vi "HFRR ADV v014 new software.vi"() -> ()   [LabVIEW 2025] (continued)
    n917 = local read "Print 3"() -> (w1079:bool)
    n918 = Equal?(x=w1076, y=path "") -> (x = y?=w1075:bool)
    n919 = Not(x=w1075) -> (.not. x?=w1074:bool)
    n920 = property on="Print 3" class="Bool (strict)"("Visible"=w1074) -> ()  [unwired: 2 in, 2 out]
    n921 = case shown="True" w1079 {
      frame False {
        n922 = local write "Rd"(TRUE ("Boolean 7")) -> ()
      }
      frame True {
        n923 = flat-sequence {
          tunnel: [w1119] -> w1087
          tunnel: [w1106] -> w1085
          tunnel: [w1116] -> w1081
          tunnel: w1087 -> [w1128]
          tunnel: [w1128] -> w1086
          tunnel: w1085 -> [w1127]
          tunnel: [w1127] -> w1084
          tunnel: [w1125] -> w1083
          tunnel: [w1124] -> w1082
          tunnel: w1081 -> [w1124]
          tunnel: w1086 -> [w1130]
          tunnel: w1084 -> [w1131]
          tunnel: w1083 -> [_]
          tunnel: w1082 -> [w1129]
          frame #0 {
            n924 = case shown="True" "Rd" {
              frame False {
              }
              frame True {
                n925 = while {
                  tunnel: "abcdefABCDEF" ("string 2") -> [w1098]
                  shift-right: [w1096] -> w1090
                  shift-left: "" -> [w1095]
                  i -> [w1105]
                  stop <- w1104 stop-if-true
                  n926 = Random Number (0-1)() -> (number: 0 to 1=w1099:dbl)
                  n927 = Multiply(x=w1099, y=62.0) -> (x*y=w1101:dbl)
                  n928 = Decrement(x="Length 2") -> (x-1=w1094:i16)
                  n929 = To Word Integer(number=w1101) -> (16bit integer=w1102:i16)
                  n930 = String Subset(string=w1098, offset (0)=w1102, length (rest)=1 ("length (rest)")) -> (substring=w1097:string)
                  n931 = Greater Or Equal?(x=w1105, y=w1094) -> (x >= y?=w1104:bool)
                  n932 = Concatenate Strings(w1097, w1095) -> (w1096:string)
                }
                "String 10" <- w1090
                n933 = local write "Rd"(FALSE ("Boolean 7")) -> ()
              }
            }
          }
          frame #1 {
            w1117 = "_resized.jpg" ("command line")
            (unwired) ".jpg -resize 320x240 " ("string")
            (unwired) "Choose an Image File" ("prompt")
            # "-resize 1798x425"
            n934 = local read "Image Path"() -> (w1111:path)
            n935 = Strip Path(path=w1111) -> (stripped path=w1106:path, name=w1107:string)
            n936 = Match Pattern(string=w1107, regular expression=".jpg") -> (before substring=→"before substring 2":string, after substring=→"after substring":string)  [unwired: 1 in, 2 out]
            n937 = Match Pattern(string=w1107, regular expression="\\") -> (before substring=w1113:string)  [unwired: 1 in, 3 out]
            n938 = Match Pattern(string=w1113, regular expression=".jpg") -> (before substring=w1112:string)  [unwired: 1 in, 3 out]
            n939 = Concatenate Strings("cmd /c convert " ("string"), w1112, ".jpg -resize 320x240  " ("command line"), w1112, w1117) -> (w1120:string)
            n940 = call <vilib>:"System Exec.vi"("run minimized? (F)"=TRUE, "wait until completion? (T)"=TRUE, "working directory"=w1106, "command line"=w1120) -> ("error out"=w1119:errorcluster)  [unwired: 4 in, 3 out]
            "error out 2" <- w1119
            n941 = Concatenate Strings(w1112, w1117) -> (w1116:string)
          }
          frame #2 {
            n942 = Wait (ms)(milliseconds to wait=u32 2000 ("millisecond timer value")) -> (millisecond timer value=w1125:u32)
          }
          frame #3 {
            n943 = case shown="No Error" w1130 {
              tunnel: w1131 -> [w1134 _]
              tunnel: w1129 -> [w1132 _]
              frame No Error {
                (unwired) ".jpg" ("string")
                n944 = Path To String(path=w1134) -> (string=w1138:string)
                n945 = Concatenate Strings(w1138, "\\" ("string"), w1132) -> (w1137:string)
                n946 = String To Path(string=w1137) -> (path=w1136:path)
                n947 = call <vilib>:"Read JPEG File.vi"("path to JPEG file"=w1136) -> ("image data"=w1140:T16)  [unwired: 8 in, 2 out]
                "image data" <- w1140
                n948 = local write "Print 3"(FALSE ("Print 2")) -> ()
                n949 = call <vilib>:"Draw Flattened Pixmap.vi"("image data"=w1140) -> ("new picture"=→"new picture":picture)  [unwired: 8 in]
              }
              frame Error {
              }
            }
          }
        }
      }
    }
    n950 = Wait (ms)(milliseconds to wait=u32 20 ("millisecond timer value")) -> ()  [unwired: 1 out]
    n951 = local read "Quit"() -> (w1073:bool)
  }
  n952 = while {
    tunnel: w33 -> [_]
    tunnel: w17 -> [_]
    stop <- w1171 stop-if-true
    # "New Adv Logics"
    n953 = local read "Main Tab"() -> (w1151:T2)
    n954 = local read "Main Tab"() -> (w1169:T2)
    n955 = local read "Sign In"() -> (w1168:bool)
    n956 = case shown="\"Adv Scar\"" w1151 {
      frame "HOME", Default {
        n957 = local read "LIVE FEED MIN TEMP"() -> (w1304:bool)
        n958 = local write "LIVE FEED MAX TEMP"(TRUE ("LIVE FEED MAX TEMP")) -> ()
        n959 = local read "CAMERA ROI MIN TEMP"() -> (w1302:bool)
        n960 = case shown="True" w1304 {
          selector: w1304 -> [_ w1311]
          frame False {
          }
          frame True {
            n961 = Not(x=w1311) -> (.not. x?=w1310:bool)
            n962 = local write "LIVE FEED MIN TEMP"(w1310) -> ()
            n963 = call "CAMERA LIVE FEED FGV.vi"("Enum - Menu"=CAMERA_LIVE_FEED_ENUM."CAMERA MINIMIZE") -> ()  [unwired: 9 in, 2 out]
          }
        }
        n964 = case shown="True" w1302 {
          selector: w1302 -> [_ w1308]
          frame False {
          }
          frame True {
            n965 = Not(x=w1308) -> (.not. x?=w1307:bool)
            n966 = local write "CAMERA ROI MIN TEMP"(w1307) -> ()
            n967 = call "IMAGE ANALYSIS.vi"("Enum"=POST_ANALYSIS_ENUM."MINIMIZE UI") -> ()  [unwired: 9 in, 2 out]
          }
        }
        n968 = local write "CAMERA ROI MAX TEMP"(TRUE ("CAMERA ROI MAX TEMP")) -> ()
      }
      frame "Test Setup" {
        n969 = local read "LIVE FEED MIN TEMP"() -> (w1314:bool)
        n970 = local read "CAMERA ROI MIN TEMP"() -> (w1312:bool)
        n971 = local write "LIVE FEED MAX TEMP"(TRUE ("LIVE FEED MAX TEMP")) -> ()
        n972 = case shown="True" w1314 {
          selector: w1314 -> [_ w1321]
          frame False {
          }
          frame True {
            n973 = Not(x=w1321) -> (.not. x?=w1320:bool)
            n974 = local write "LIVE FEED MIN TEMP"(w1320) -> ()
            n975 = call "CAMERA LIVE FEED FGV.vi"("Enum - Menu"=CAMERA_LIVE_FEED_ENUM."CAMERA MINIMIZE") -> ()  [unwired: 9 in, 2 out]
          }
        }
        n976 = case shown="True" w1312 {
          selector: w1312 -> [_ w1318]
          frame False {
          }
          frame True {
            n977 = Not(x=w1318) -> (.not. x?=w1317:bool)
            n978 = local write "CAMERA ROI MIN TEMP"(w1317) -> ()
            n979 = call "IMAGE ANALYSIS.vi"("Enum"=POST_ANALYSIS_ENUM."MINIMIZE UI") -> ()  [unwired: 9 in, 2 out]
          }
        }
        n980 = local write "CAMERA ROI MAX TEMP"(TRUE ("CAMERA ROI MAX TEMP")) -> ()
      }
      frame "Acquire" {
        n981 = local read "LIVE FEED MIN TEMP"() -> (w1324:bool)
        n982 = local write "LIVE FEED MAX TEMP"(TRUE ("LIVE FEED MAX TEMP")) -> ()
        n983 = local read "CAMERA ROI MIN TEMP"() -> (w1322:bool)
        n984 = case shown="True" w1324 {
          selector: w1324 -> [_ w1331]
          frame False {
          }
          frame True {
            n985 = Not(x=w1331) -> (.not. x?=w1330:bool)
            n986 = local write "LIVE FEED MIN TEMP"(w1330) -> ()
            n987 = call "CAMERA LIVE FEED FGV.vi"("Enum - Menu"=CAMERA_LIVE_FEED_ENUM."CAMERA MINIMIZE") -> ()  [unwired: 9 in, 2 out]
          }
        }
        n988 = case shown="True" w1322 {
          selector: w1322 -> [_ w1328]
          frame False {
          }
          frame True {
            n989 = Not(x=w1328) -> (.not. x?=w1327:bool)
            n990 = local write "CAMERA ROI MIN TEMP"(w1327) -> ()
            n991 = call "IMAGE ANALYSIS.vi"("Enum"=POST_ANALYSIS_ENUM."MINIMIZE UI") -> ()  [unwired: 9 in, 2 out]
          }
        }
        n992 = local write "CAMERA ROI MAX TEMP"(TRUE ("CAMERA ROI MAX TEMP")) -> ()
      }
      frame "Adv Scar" {
        n993 = local read "CAMERA ROI MIN TEMP"() -> (w1332:bool)
        n994 = case shown="True" "LIVE FEED MAX TEMP" {
          selector: "LIVE FEED MAX TEMP" -> [_ w1353]
          frame False {
          }
          frame True {
            n995 = Not(x=w1353) -> (.not. x?=w1352:bool)
            n996 = local write "LIVE FEED MAX TEMP"(w1352) -> ()
            n997 = call "CAMERA LIVE FEED FGV.vi"("Enum - Menu"=CAMERA_LIVE_FEED_ENUM."CAMERA RESTORE") -> ("error out"=w1343:errorcluster)  [unwired: 9 in, 1 out]
            n998 = Type Cast(type=30, x=0) -> (*(type *) &x=w1347:i32)
            n999 = Add(x=w1347, y=48) -> (x+y=w1348:i32)
            n1000 = call "CAMERA LIVE FEED FGV.vi"("Enum - Menu"=CAMERA_LIVE_FEED_ENUM."CAMERA MODE SET", "error in (no error)"=w1343, "CAMERA MODE"=w1348) -> ("error out"=w1340:errorcluster)  [unwired: 7 in, 1 out]
            n1001 = call "CAMERA LIVE FEED FGV.vi"("Enum - Menu"=CAMERA_LIVE_FEED_ENUM."CAMERA GRAY", "error in (no error)"=w1340) -> ("error out"=w1339:errorcluster)  [unwired: 8 in, 1 out]
            n1002 = call "LIST FILE NAMES.vi"("error in (no error)"=w1339) -> ("error out"=w1349:errorcluster, "filenames"=w1350:string[])  [unwired: 9 in]
            n1003 = property on="FILE 3" class="CmbBox"(error in=w1349, "Strings[]"=w1350) -> ()  [unwired: 1 in, 2 out]
          }
        }
        n1004 = case shown="True" w1332 {
          selector: w1332 -> [_ w1338]
          frame False {
          }
          frame True {
            n1005 = Not(x=w1338) -> (.not. x?=w1337:bool)
            n1006 = local write "CAMERA ROI MIN TEMP"(w1337) -> ()
            n1007 = call "IMAGE ANALYSIS.vi"("Enum"=POST_ANALYSIS_ENUM."MINIMIZE UI") -> ()  [unwired: 9 in, 2 out]
          }
        }
        n1008 = local write "CAMERA ROI MAX TEMP"(TRUE ("CAMERA ROI MAX TEMP")) -> ()
        "LIVE FEED MIN TEMP" <- TRUE ("LIVE FEED MIN TEMP")
      }
      frame "Adv Scar Report" {
        n1009 = local read "CAMERA ROI MAX TEMP"() -> (w1354:bool)
        n1010 = local read "LIVE FEED MIN TEMP"() -> (w1356:bool)
        n1011 = local write "LIVE FEED MAX TEMP"(TRUE ("LIVE FEED MAX TEMP")) -> ()
        n1012 = case shown="True" w1356 {
          selector: w1356 -> [_ w1365]
          frame False {
          }
          frame True {
            n1013 = Not(x=w1365) -> (.not. x?=w1364:bool)
            n1014 = local write "LIVE FEED MIN TEMP"(w1364) -> ()
            n1015 = call "CAMERA LIVE FEED FGV.vi"("Enum - Menu"=CAMERA_LIVE_FEED_ENUM."CAMERA MINIMIZE") -> ()  [unwired: 9 in, 2 out]
          }
        }
        n1016 = case shown="True" w1354 {
          selector: w1354 -> [_ w1362]
          frame False {
          }
          frame True {
            n1017 = Not(x=w1362) -> (.not. x?=w1360:bool)
            n1018 = local write "CAMERA ROI MAX TEMP"(w1360) -> ()
            n1019 = call "IMAGE ANALYSIS.vi"("Enum"=POST_ANALYSIS_ENUM."SHOW UI") -> ("error out"=w1359:errorcluster)  [unwired: 9 in, 1 out]
            n1020 = call "LIST FILE NAMES.vi"("error in (no error)"=w1359) -> ("filenames"=w1358:string[])  [unwired: 9 in, 1 out]
            n1021 = property on="Test File List :" class="CmbBox"("Strings[]"=w1358) -> ()  [unwired: 2 in, 2 out]
          }
        }
        n1022 = local write "CAMERA ROI MIN TEMP"(TRUE ("CAMERA ROI MIN TEMP")) -> ()
      }
      frame "Compare Files" {
        n1023 = local read "LIVE FEED MIN TEMP"() -> (w1368:bool)
        n1024 = local write "LIVE FEED MAX TEMP"(TRUE ("LIVE FEED MAX TEMP")) -> ()
        n1025 = local read "CAMERA ROI MIN TEMP"() -> (w1366:bool)
        n1026 = case shown="True" w1368 {
          selector: w1368 -> [_ w1375]
          frame False {
          }
          frame True {
            n1027 = Not(x=w1375) -> (.not. x?=w1374:bool)
            n1028 = local write "LIVE FEED MIN TEMP"(w1374) -> ()
            n1029 = call "CAMERA LIVE FEED FGV.vi"("Enum - Menu"=CAMERA_LIVE_FEED_ENUM."CAMERA MINIMIZE") -> ()  [unwired: 9 in, 2 out]
          }
        }
        n1030 = case shown="True" w1366 {
          selector: w1366 -> [_ w1372]
          frame False {
          }
          frame True {
            n1031 = Not(x=w1372) -> (.not. x?=w1371:bool)
            n1032 = local write "CAMERA ROI MIN TEMP"(w1371) -> ()
            n1033 = call "IMAGE ANALYSIS.vi"("Enum"=POST_ANALYSIS_ENUM."MINIMIZE UI") -> ()  [unwired: 9 in, 2 out]
          }
        }
        n1034 = local write "CAMERA ROI MAX TEMP"(TRUE ("CAMERA ROI MAX TEMP")) -> ()
      }
      frame "About" {
        n1035 = local read "LIVE FEED MIN TEMP"() -> (w1378:bool)
        n1036 = local write "LIVE FEED MAX TEMP"(TRUE ("LIVE FEED MAX TEMP")) -> ()
        n1037 = local read "CAMERA ROI MIN TEMP"() -> (w1377:bool)
        n1038 = case shown="True" w1378 {
          selector: w1378 -> [_ w1385]
          frame False {
          }
          frame True {
            n1039 = Not(x=w1385) -> (.not. x?=w1384:bool)
            n1040 = local write "LIVE FEED MIN TEMP"(w1384) -> ()
            n1041 = call "CAMERA LIVE FEED FGV.vi"("Enum - Menu"=CAMERA_LIVE_FEED_ENUM."CAMERA MINIMIZE") -> ()  [unwired: 9 in, 2 out]
          }
        }
        n1042 = case shown="True" w1377 {
          selector: w1377 -> [_ w1382]
          frame False {
          }
          frame True {
            n1043 = Not(x=w1382) -> (.not. x?=w1381:bool)
            n1044 = local write "CAMERA ROI MIN TEMP"(w1381) -> ()
            n1045 = call "IMAGE ANALYSIS.vi"("Enum"=POST_ANALYSIS_ENUM."MINIMIZE UI") -> ()  [unwired: 9 in, 2 out]
          }
        }
        n1046 = local write "CAMERA ROI MAX TEMP"(TRUE ("CAMERA ROI MIN TEMP")) -> ()
      }
      frame "Advance" {
        n1047 = local read "LIVE FEED MIN TEMP"() -> (w1388:bool)
        n1048 = local write "LIVE FEED MAX TEMP"(TRUE ("LIVE FEED MAX TEMP")) -> ()
        n1049 = local read "CAMERA ROI MIN TEMP"() -> (w1386:bool)
        n1050 = case shown="True" w1388 {
          selector: w1388 -> [_ w1395]
          frame False {
          }
          frame True {
            n1051 = Not(x=w1395) -> (.not. x?=w1394:bool)
            n1052 = local write "LIVE FEED MIN TEMP"(w1394) -> ()
            n1053 = call "CAMERA LIVE FEED FGV.vi"("Enum - Menu"=CAMERA_LIVE_FEED_ENUM."CAMERA MINIMIZE") -> ()  [unwired: 9 in, 2 out]
          }
        }
        n1054 = local write "CAMERA ROI MAX TEMP"(TRUE ("CAMERA ROI MAX TEMP")) -> ()
        n1055 = case shown="True" w1386 {
          selector: w1386 -> [_ w1392]
          frame False {
          }
          frame True {
            n1056 = Not(x=w1392) -> (.not. x?=w1391:bool)
            n1057 = local write "CAMERA ROI MIN TEMP"(w1391) -> ()
            n1058 = call "IMAGE ANALYSIS.vi"("Enum"=POST_ANALYSIS_ENUM."MINIMIZE UI") -> ()  [unwired: 9 in, 2 out]
          }
        }
      }
      frame "Mooha" {
        n1059 = local read "LIVE FEED MIN TEMP"() -> (w1398:bool)
        n1060 = local write "LIVE FEED MAX TEMP"(TRUE ("LIVE FEED MAX TEMP")) -> ()
        n1061 = local read "CAMERA ROI MIN TEMP"() -> (w1396:bool)
        n1062 = case shown="True" w1398 {
          selector: w1398 -> [_ w1405]
          frame False {
          }
          frame True {
            n1063 = Not(x=w1405) -> (.not. x?=w1404:bool)
            n1064 = local write "LIVE FEED MIN TEMP"(w1404) -> ()
            n1065 = call "CAMERA LIVE FEED FGV.vi"("Enum - Menu"=CAMERA_LIVE_FEED_ENUM."CAMERA MINIMIZE") -> ()  [unwired: 9 in, 2 out]
          }
        }
        n1066 = local write "CAMERA ROI MAX TEMP"(TRUE ("CAMERA ROI MAX TEMP")) -> ()
        n1067 = case shown="True" w1396 {
          selector: w1396 -> [_ w1402]
          frame False {
          }
          frame True {
            n1068 = Not(x=w1402) -> (.not. x?=w1401:bool)
            n1069 = local write "CAMERA ROI MIN TEMP"(w1401) -> ()
            n1070 = call "IMAGE ANALYSIS.vi"("Enum"=POST_ANALYSIS_ENUM."MINIMIZE UI") -> ()  [unwired: 9 in, 2 out]
          }
        }
      }
    }
    n1071 = local read "Auto Start Test"() -> (w1142:bool)
    n1072 = case shown="True" "sign in temp" {
      frame False {
      }
      frame True {
        w1178 = 1 ("y")
        n1073 = local read "USERNAME"() -> (w1184:string)
        n1074 = local read "USER ID"() -> (w1181:string)
        n1075 = call <vilib>:"Trim Whitespace.vi"("string"=w1184) -> ("trimmed string"=w1183:string)  [unwired: 1 in]
        n1076 = call <vilib>:"Trim Whitespace.vi"("string"=w1181) -> ("trimmed string"=w1182:string)  [unwired: 1 in]
        n1077 = String Length(string=w1183) -> (length=w1180:i32)
        n1078 = String Length(string=w1182) -> (length=w1179:i32)
        n1079 = Greater?(x=w1180, y=w1178) -> (0:w1177:bool)
        n1080 = Greater?(x=w1179, y=w1178) -> (0:w1176:bool)
        n1081 = And(x=w1177, y=w1176) -> (x .and. y?=w1175:bool)
        n1082 = case shown="True" w1175 {
          frame False {
            n1083 = property on="Sign In" class="Bool (strict)"("DisabledEnum"=T18."Disabled" ("Disabled")) -> ()  [unwired: 2 in, 2 out]
          }
          frame True {
            n1084 = property on="Sign In" class="Bool (strict)"("DisabledEnum"=T18."Enabled" ("Disabled")) -> ()  [unwired: 2 in, 2 out]
          }
        }
      }
    }
    n1085 = local read "Air Temperature"() -> (w1159:bool)
    n1086 = local read "Coefficient Of Friction"() -> (w1160:bool)
    n1087 = case shown="False" w1142 {
      frame False {
        n1088 = local read "Auto stop temp"() -> (w1172:bool)
        n1089 = case shown="True" w1172 {
          frame False {
          }
          frame True {
            n1090 = local write "Auto Start Temp"(FALSE ("Auto Start Temp")) -> ()
          }
        }
      }
      frame True {
        "Auto stop temp" <- TRUE ("Auto stop temp")
      }
    }
    n1091 = local read "Humidity"() -> (w1158:bool)
    n1092 = case shown="\"HOME\"" w1169 {
      frame "HOME" {
        n1093 = local write "main tab sub"(enum32{"Page 1", "Page 2"}."Page 1" ("main tab sub")) -> ()
      }
      frame Default {
        n1094 = local write "main tab sub"(enum32{"Page 1", "Page 2"}."Page 2" ("main tab sub")) -> ()
      }
    }
    n1095 = case shown="True" w1168 {
      selector: w1168 -> [_ w1519]
      frame False {
      }
      frame True {
        n1096 = Not(x=w1519) -> (.not. x?=w1518:bool)
        n1097 = local write "Sign In"(w1518) -> ()
        n1098 = local write "Main Dashboard Buttons"(T24."Test Setup" ("Main Dashboard Buttons")) -> ()
      }
    }
    n1099 = case shown="\"Numeric Display\", Default" "Num/Graph" {
      frame "Numeric Display", Default {
        n1100 = property on="Single/Multiple" class="RadioBtnsControl (strict)"("Visible"=FALSE) -> ()  [unwired: 2 in, 2 out]
        n1101 = property on="Single - Graph" class="Ring (strict)"("Visible"=FALSE) -> ()  [unwired: 2 in, 2 out]
        n1102 = local write "Main Tab Display"(T4."Dashboard 1" ("Main Tab Display")) -> ()
      }
      frame "Graph Display" {
        n1103 = property on="Single/Multiple" class="RadioBtnsControl (strict)"("Visible"=TRUE) -> ()  [unwired: 2 in, 2 out]
        n1104 = case shown="\"Multiple\"" "Single/Multiple" {
          frame "Single ", Default {
            n1105 = property on="Single - Graph" class="Ring (strict)"("Visible"=TRUE) -> ()  [unwired: 2 in, 2 out]
            n1106 = local write "Main Tab Display"(T4."Dashboard 3" ("Main Tab Display")) -> ()
          }
          frame "Multiple" {
            n1107 = property on="Single - Graph" class="Ring (strict)"("Visible"=FALSE) -> ()  [unwired: 2 in, 2 out]
            n1108 = local write "Main Tab Display"(T4."Dashboard 2" ("Main Tab Display")) -> ()
          }
        }
      }
    }
    n1109 = local read "Stroke"() -> (w1157:bool)
    n1110 = local read "USERNAME"() -> (w1163:string)
    n1111 = local read "USER ID"() -> (w1162:string)
    n1112 = case shown="True" w1160 {
      selector: w1160 -> [_ w1445]
      frame False {
      }
      frame True {
        n1113 = Not(x=w1445) -> (.not. x?=w1444:bool)
        n1114 = local write "Coefficient Of Friction"(w1444) -> ()
        n1115 = local write "Tab Control 2"(T6."Coefficient Of Friction" ("Tab Control 2")) -> ()
      }
    }
    n1116 = case shown="True" w1159 {
      selector: w1159 -> [_ w1442]
      frame False {
      }
      frame True {
        n1117 = Not(x=w1442) -> (.not. x?=w1440:bool)
        n1118 = local write "Air Temperature"(w1440) -> ()
        n1119 = local write "Tab Control 2"(T6."Air Temperature" ("Tab Control 2")) -> ()
      }
    }
    n1120 = local write "Operator ID"(w1162) -> ()
    n1121 = case shown="True" w1157 {
      selector: w1157 -> [_ w1436]
      frame False {
      }
      frame True {
        n1122 = Not(x=w1436) -> (.not. x?=w1434:bool)
        n1123 = local write "Stroke"(w1434) -> ()
        n1124 = local write "Tab Control 2"(T6."Stroke" ("Tab Control 2")) -> ()
      }
    }
    n1125 = local write "tested by"(w1163) -> ()
    n1126 = case shown="True" w1158 {
      selector: w1158 -> [_ w1439]
      frame False {
      }
      frame True {
        n1127 = Not(x=w1439) -> (.not. x?=w1437:bool)
        n1128 = local write "Humidity"(w1437) -> ()
        n1129 = local write "Tab Control 2"(T6."Humidity" ("Tab Control 2")) -> ()
      }
    }
    n1130 = case shown="\"Calibration\"" "Main Dashboard Buttons" {
      tunnel: [T2."HOME" ("Main Tab") T2."Test Setup" ("Main Tab") T2."Acquire" ("Main Tab") T2."Adv Scar" ("Main Tab") T2."Adv Scar Report" ("Main Tab") T2."Compare Files" ("Main Tab") T2."Calibration" ("Main Tab") T2."About" ("Main Tab") T2."Advance" ("Main Tab")] -> w1141
      frame "Home", Default {
      }
      frame "Test Setup" {
      }
      frame "Dashboard" {
      }
      frame "Imaging" {
      }
      frame "Report" {
      }
      frame "Analysis" {
      }
      frame "Calibration" {
      }
      frame "About" {
      }
      frame "Advance" {
      }
    }
    n1131 = Wait (ms)(milliseconds to wait=u32 100) -> ()  [unwired: 1 out]
    n1132 = local read "Main Tab Display"() -> (w1161:T4)
    n1133 = local write "Main Tab"(w1141) -> ()
    n1134 = case shown="\"Dashboard 3\"" w1161 {
      frame "Dashboard 1", Default {
        n1135 = property on="Reset Graph" class="Bool (strict)"("Visible"=FALSE) -> ()  [unwired: 2 in, 2 out]
      }
      frame "Dashboard 2" {
        n1136 = property on="Reset Graph" class="Bool (strict)"("Visible"=TRUE) -> ()  [unwired: 2 in, 2 out]
      }
      frame "Dashboard 3" {
        n1137 = property on="Reset Graph" class="Bool (strict)"("Visible"=TRUE) -> ()  [unwired: 2 in, 2 out]
      }
    }
    n1138 = local read "SCAR MEASURMENT"() -> (w1149:enum32{"Auto Scar", "Manual Scar"})
    n1139 = local read "Humidity"() -> (w1164:bool)
    n1140 = local read "Cap Live Image"() -> (w1146:bool)
    n1141 = local read "Sample Temperature"() -> (w1156:bool)
    n1142 = local read "Air Temp vs Humidity"() -> (w1154:bool)
    n1143 = local read "Frequency"() -> (w1155:bool)
    n1144 = case shown="True" w1164 {
      frame False {
        n1145 = local write "Humidity On Command"(TRUE ("Humidity On Command")) -> ()
        n1146 = case shown="True" "Humidity Off Command" {
          selector: "Humidity Off Command" -> [_ w1452]
          frame False {
          }
          frame True {
            n1147 = stacked-sequence {
              frame #0 {
                n1148 = local read "WriteHumidity"() -> (w1454:string[])
                n1149 = Insert Into Array(array=w1454, new element="R;1" ("new element/subarray")) -> (w1455:string[])  [unwired: 1 in]
                n1150 = local write "WriteHumidity"(w1455) -> ()
              }
              frame #1 {
                n1151 = Wait (ms)(milliseconds to wait=u32 2000) -> ()  [unwired: 1 out]
              }
              frame #2 {
                n1152 = local read "EVENT LOG"() -> (w1461:string)
                n1153 = local read "WriteHumidity"() -> (w1458:string[])
                n1154 = call "Event Log.vi"("Content"="Humidity Control Off" ("string"), "EVENT LOG"=w1461) -> ("EVENT LOG"=w1462:string)  [unwired: 8 in, 1 out]
                n1155 = local write "EVENT LOG"(w1462) -> ()
                n1156 = Insert Into Array(array=w1458, new element="R;1" ("new element/subarray")) -> (w1459:string[])  [unwired: 1 in]
                n1157 = local write "WriteHumidity"(w1459) -> ()
              }
            }
            n1158 = Not(x=w1452) -> (.not. x?=w1451:bool)
            n1159 = local write "Humidity Off Command"(w1451) -> ()
          }
        }
      }
      frame True {
        n1160 = local write "Humidity Off Command"(TRUE ("Humidity Off Command")) -> ()
        n1161 = case shown="True" "Humidity On Command" {
          selector: "Humidity On Command" -> [_ w1466]
          frame False {
          }
          frame True {
            n1162 = stacked-sequence {
              frame #0 {
                n1163 = local read "Set Rh"() -> (w1472:dbl)
                n1164 = Number To Fractional String(number=w1472, precision (6)=i16 2) -> (F-format string=w1473:string)  [unwired: 2 in]
                n1165 = local read "WriteHumidity"() -> (w1470:string[])
                n1166 = Concatenate Strings("M;" ("new element/subarray"), w1473) -> (w1471:string)
                n1167 = Insert Into Array(array=w1470, new element=w1471) -> (w1469:string[])  [unwired: 1 in]
                n1168 = local write "WriteHumidity"(w1469) -> ()
              }
              frame #1 {
                n1169 = Wait (ms)(milliseconds to wait=u32 2000) -> ()  [unwired: 1 out]
              }
              frame #2 {
                n1170 = local read "Set Rh"() -> (w1480:dbl)
                n1171 = Number To Fractional String(number=w1480, precision (6)=i16 2) -> (F-format string=w1481:string)  [unwired: 2 in]
                n1172 = local read "WriteHumidity"() -> (w1478:string[])
                n1173 = Concatenate Strings("M;" ("new element/subarray"), w1481) -> (w1479:string)
                n1174 = Insert Into Array(array=w1478, new element=w1479) -> (w1477:string[])  [unwired: 1 in]
                n1175 = local write "WriteHumidity"(w1477) -> ()
              }
              frame #3 {
                n1176 = Wait (ms)(milliseconds to wait=u32 1500) -> ()  [unwired: 1 out]
              }
              frame #4 {
                (unwired) "% RH" ("string")
                (unwired) i16 2 ("precision (6)")
                (unwired) "M;" ("new element/subarray")
                n1177 = local read "Set Rh"() -> (w1488:dbl)
                n1178 = Number To Fractional String(number=w1488, precision (6)=i16 2) -> (F-format string=w1485:string)  [unwired: 2 in]
                n1179 = local read "WriteHumidity"() -> (w1490:string[])
                n1180 = Concatenate Strings("M;" ("new element/subarray"), w1485) -> (w1489:string)
                n1181 = Concatenate Strings("Humidity Set to : " ("string"), w1485, "% RH" ("string")) -> (w1483:string)
                n1182 = Insert Into Array(array=w1490, new element=w1489) -> (w1491:string[])  [unwired: 1 in]
                n1183 = disable-structure shown="Enabled" {
                  frame Enabled {
                    n1184 = local read "EVENT LOG"() -> (w1494:string)
                    n1185 = call "Event Log.vi"("Content"="Humidity Control On", "EVENT LOG"=w1494) -> ("EVENT LOG"=w1495:string)  [unwired: 8 in, 1 out]
                    n1186 = local write "EVENT LOG"(w1495) -> ()
                  }
                  frame Disabled {
                  }
                }
                n1187 = disable-structure shown="Enabled" {
                  disable-tunnel: w1483 -> [_ _]
                  frame Enabled {
                    n1188 = local read "EVENT LOG"() -> (w1497:string)
                    n1189 = call "Event Log.vi"("Content"="Humidity Control On", "EVENT LOG"=w1497) -> ("EVENT LOG"=w1498:string)  [unwired: 8 in, 1 out]
                    n1190 = local write "EVENT LOG"(w1498) -> ()
                  }
                  frame Disabled {
                  }
                }
                n1191 = local write "WriteHumidity"(w1491) -> ()
              }
            }
            n1192 = Not(x=w1466) -> (.not. x?=w1465:bool)
            n1193 = local write "Humidity On Command"(w1465) -> ()
          }
        }
      }
    }
    n1194 = Equal?(x=w1149, y=enum32{"Auto Scar", "Manual Scar"}."Auto Scar" ("SCAR MEASURMENT")) -> (x = y?=w1145:bool)
    n1195 = local read "TEST STANDARD"() -> (w1152:T3)
    n1196 = And(x=w1146, y=w1145) -> (x .and. y?=w1147:bool)
    n1197 = case shown="True" w1147 {
      selector: w1147 -> [_ w1251]
      tunnel: errorcluster {"status"=FALSE, "code"=0, "source"=""} ("error in (no error) 3") -> [_ w1252]
      frame False {
      }
      frame True {
        n1198 = stacked-sequence {
          tunnel: w1252 -> [_ _ _ _ _ _ _ w1300]
          tunnel: w1251 -> [_ _ _ _ _ w1281 _ _]
          frame #0 {
            n1199 = call "CAMERA LIVE FEED FGV.vi"("Enum - Menu"=CAMERA_LIVE_FEED_ENUM."CAMERA MINIMIZE") -> ()  [unwired: 9 in, 2 out]
          }
          frame #1 {
            n1200 = property on="Auto Scar Check  2" class="Clust (strict)"("Visible"=TRUE) -> ()  [unwired: 2 in, 2 out]
          }
          frame #2 {
            n1201 = String To Path(string="C:\\LAB-IQ\\Image Calibrate v01.dcf") -> (path=w1257:path)
            n1202 = Open/Create/Replace File ("Open File")(file path (use dialog)=w1257) -> (refnum out=w1258:refnum<file>)  [unwired: 5 in, 2 out]
            n1203 = for {
              N: 4 -> [_]
              tunnel: w1258 -> [w1264]
              i -> [w1260]
              n1204 = Read from Text File ("Read File")(file (use dialog)=w1264) -> (text=w1265:string)  [unwired: 3 in, 3 out]
              n1205 = String Subset(string=w1265, offset (0)=6, length (rest)=10 ("length (rest)")) -> (substring=w1261:string)
              n1206 = Fract/Exp String To Number(string=w1261) -> (number=w1259:dbl)  [unwired: 3 in, 1 out]
              n1207 = case shown="0" w1260 {
                tunnel: w1259 -> [w1266 w1267 _ w1268 _]
                frame 0 {
                  "5x Gain" <- w1266
                }
                frame 1 {
                  "10x Gain" <- w1267
                }
                frame 2 {
                }
                frame 3 {
                  "100x gain" <- w1268
                }
                frame 4, Default {
                }
              }
            }
          }
          frame #3 {
            n1208 = local read "FILE 3"() -> (w1274:string)
            n1209 = call <vilib>:"Trim Whitespace.vi"("string"="C:\\LAB-IQ\\images\\") -> ("trimmed string"=w1276:string)  [unwired: 1 in]
            n1210 = String To Path(string=w1276) -> (path=w1275:path)
            n1211 = Concatenate Strings(w1274, ".png" ("string")) -> (w1273:string)
            n1212 = Build Path(base path=w1275, name or relative path=w1273) -> (appended path=w1271:path)
            "Image path" <- w1271
            n1213 = Path To String(path=w1271) -> (string=w1270:string)
            n1214 = call "CAMERA LIVE FEED FGV.vi"("Enum - Menu"=CAMERA_LIVE_FEED_ENUM."CAMERA SAVE", "Image Path"=w1270) -> ()  [unwired: 8 in, 2 out]
          }
          frame #4 {
            n1215 = One Button Dialog(message="Image saved successfully") -> ()  [unwired: 1 in, 1 out]
          }
          frame #5 {
            n1216 = local read "TEST STANDARD"() -> (w1280:T3)
            n1217 = local read "Magnification len live scar"() -> (w1292:string)
            n1218 = Not(x=w1281) -> (.not. x?=w1282:bool)
            n1219 = local write "Cap Live Image"(w1282) -> ()
            n1220 = case shown="\"ISO 12156\"" w1280 {
              tunnel: ["ASTM D6079" "ISO 12156"] -> w1279
              frame "ASTM D6079", Default {
              }
              frame "ISO 12156" {
              }
            }
            n1221 = case shown="\"5x\", Default" w1292 {
              tunnel: [w1295 w1296] -> w1291
              frame "5x", Default {
                n1222 = local read "5x Gain"() -> (w1295:dbl)
              }
              frame "10x" {
                # "5x"
                n1223 = local read "10x Gain"() -> (w1296:dbl)
              }
            }
            n1224 = local read "Image path"() -> (w1290:path)
            n1225 = local read "FILE 3"() -> (w1283:string)
            n1226 = call "EDGE DETCTION.vi"("GAIN VALUE"=w1291, "Image Path"=w1290) -> ("error out"=w1289:errorcluster, "return value"=w1288:cluster{string, string, dbl, dbl, dbl})  [unwired: 8 in]
            n1227 = Bundle By Name(cluster=T25 {"File Name"="", "Test Method"="", "Operator"="", "Fuel Description"="", "Date and time"=""} ("Main Ref"), "File Name"=w1283, "Test Method"=w1279) -> (w1284:T25)
            n1228 = call "duf file read.vi"("error in (no error)"=w1289, "Main Ref"=w1284) -> ("error out"=w1287:errorcluster, "Main Ref 2"=w1285:T25)  [unwired: 8 in]
            n1229 = call "EDGE DETECTION REPORT.vi"("error in (no error)"=w1287, "return value 2"=w1288, "Main Ref"=w1285) -> ()  [unwired: 8 in, 1 out]
          }
          frame #6 {
            n1230 = property on="Auto Scar Check  2" class="Clust (strict)"("Visible"=FALSE) -> ()  [unwired: 2 in, 2 out]
          }
          frame #7 {
            n1231 = call "CAMERA LIVE FEED FGV.vi"("Enum - Menu"=CAMERA_LIVE_FEED_ENUM."CAMERA MINIMIZE", "error in (no error)"=w1300) -> ()  [unwired: 8 in, 2 out]
            n1232 = local write "Main Dashboard Buttons"(T1."Home" ("Main Dashboard Buttons")) -> ()
            n1233 = local write "Main Tab"(T2."HOME" ("Main Tab")) -> ()
          }
        }
      }
    }
    n1234 = local read "Heater Button"() -> (w1153:bool)
    n1235 = case shown="True" w1155 {
      selector: w1155 -> [_ w1430]
      frame False {
      }
      frame True {
        n1236 = Not(x=w1430) -> (.not. x?=w1428:bool)
        n1237 = local write "Frequency"(w1428) -> ()
        n1238 = local write "Tab Control 2"(T6."Frequency" ("Tab Control 2")) -> ()
      }
    }
    n1239 = case shown="True" w1154 {
      selector: w1154 -> [_ w1427]
      frame False {
      }
      frame True {
        n1240 = Not(x=w1427) -> (.not. x?=w1425:bool)
        n1241 = local write "Air Temp vs Humidity"(w1425) -> ()
        n1242 = local write "Tab Control 2"(T6."Air Temp vs Rh" ("Tab Control 2")) -> ()
      }
    }
    n1243 = case shown="True" w1156 {
      selector: w1156 -> [_ w1433]
      frame False {
      }
      frame True {
        n1244 = Not(x=w1433) -> (.not. x?=w1431:bool)
        n1245 = local write "Sample Temperature"(w1431) -> ()
        n1246 = local write "Tab Control 2"(T6."Sample Temperature" ("Tab Control 2")) -> ()
      }
    }
    n1247 = case shown="\"Custom\"" w1152 {
      frame "ASTM D6079", Default {
        w1406 = "ASTM D6079 TEST CONDITIONS" ("Standard 2")
        n1248 = local write "Standard 2"(w1406) -> ()
        n1249 = local write "Standard"(w1406) -> ()
      }
      frame "ISO 12156" {
        w1407 = "ISO 12156 TEST CONDITIONS" ("Standard 2")
        n1250 = local write "Standard 2"(w1407) -> ()
        n1251 = local write "Standard"(w1407) -> ()
      }
      frame "CEC F-096-A-06" {
        w1408 = "CEC F-096-A-06 TEST CONDITIONS" ("Standard 2")
        n1252 = local write "Standard 2"(w1408) -> ()
        n1253 = local write "Standard"(w1408) -> ()
      }
      frame "Custom" {
        w1409 = "CUSTOM TEST CONDITIONS" ("Standard 2")
        n1254 = local write "Standard 2"(w1409) -> ()
        n1255 = local write "Standard"(w1409) -> ()
      }
    }
    n1256 = case shown="True" w1153 {
      frame False {
        n1257 = local write "Temperature On Command"(TRUE ("Temperature On Command")) -> ()
        n1258 = case shown="True" "Temperature Off Command" {
          selector: "Temperature Off Command" -> [_ w1413]
          frame False {
          }
          frame True {
            n1259 = Not(x=w1413) -> (.not. x?=w1412:bool)
            n1260 = local read "EVENT LOG"() -> (w1416:string)
            n1261 = local write "Temperature Off Command"(w1412) -> ()
            n1262 = call "Event Log.vi"("Content"="Heater Off", "EVENT LOG"=w1416) -> ("EVENT LOG"=w1415:string)  [unwired: 8 in, 1 out]
            n1263 = local write "EVENT LOG"(w1415) -> ()
          }
        }
      }
      frame True {
        n1264 = local write "Temperature Off Command"(TRUE ("Temperature Off Command")) -> ()
        n1265 = case shown="True" "Temperature On Command" {
          selector: "Temperature On Command" -> [_ w1420]
          frame False {
          }
          frame True {
            n1266 = Not(x=w1420) -> (.not. x?=w1419:bool)
            n1267 = local write "Temperature On Command"(w1419) -> ()
            n1268 = disable-structure shown="Enabled" {
              disable-tunnel: "Heater On" -> [w1422 _]
              frame Enabled {
                n1269 = local read "EVENT LOG"() -> (w1423:string)
                n1270 = call "Event Log.vi"("Content"=w1422, "EVENT LOG"=w1423) -> ("EVENT LOG"=w1424:string)  [unwired: 8 in, 1 out]
                n1271 = local write "EVENT LOG"(w1424) -> ()
              }
              frame Disabled {
              }
            }
          }
        }
      }
    }
    n1272 = local read "Main Tab"() -> (w1144:T2)
    n1273 = case shown="\"About\"" w1144 {
      frame "HOME", Default {
        w1187 = T18."Enabled" ("Disabled")
        n1274 = local read "Service Password enable"() -> (w1189:bool)
        n1275 = property on="Imaging" class="Bool (strict)"("DisabledEnum"=w1187) -> ()  [unwired: 2 in, 2 out]
        n1276 = property on="Dashboard" class="Bool (strict)"("DisabledEnum"=w1187) -> ()  [unwired: 2 in, 2 out]
        n1277 = property on="Test Setup" class="Bool (strict)"("DisabledEnum"=w1187) -> ()  [unwired: 2 in, 2 out]
        n1278 = property on="Analysis" class="Bool (strict)"("DisabledEnum"=w1187) -> ()  [unwired: 2 in, 2 out]
        n1279 = property on="Home" class="Bool (strict)"("DisabledEnum"=w1187) -> ()  [unwired: 2 in, 2 out]
        n1280 = property on="Report" class="Bool (strict)"("DisabledEnum"=w1187) -> ()  [unwired: 2 in, 2 out]
        n1281 = property on="Main Dashboard Buttons" class="RadioBtnsControl (strict)"("DisabledEnum"=w1187) -> ()  [unwired: 2 in, 2 out]
        n1282 = property on="Calibration" class="Bool (strict)"("DisabledEnum"=w1187) -> ()  [unwired: 2 in, 2 out]
        n1283 = case shown="True" w1189 {
          tunnel: [T18."Disabled" ("Disabled") T18."Enabled" ("Disabled")] -> w1188
          frame False {
          }
          frame True {
          }
        }
        n1284 = property on="About" class="Bool (strict)"("DisabledEnum"=w1188) -> ()  [unwired: 2 in, 2 out]
      }
      frame "Test Setup" {
        w1194 = T18."Enabled" ("Disabled")
        n1285 = local read "Service Password enable"() -> (w1193:bool)
        n1286 = property on="Dashboard" class="Bool (strict)"("DisabledEnum"=T18."Disabled" ("Disabled")) -> ()  [unwired: 2 in, 2 out]
        n1287 = property on="Imaging" class="Bool (strict)"("DisabledEnum"=w1194) -> ()  [unwired: 2 in, 2 out]
        n1288 = property on="Analysis" class="Bool (strict)"("DisabledEnum"=w1194) -> ()  [unwired: 2 in, 2 out]
        n1289 = property on="Home" class="Bool (strict)"("DisabledEnum"=w1194) -> ()  [unwired: 2 in, 2 out]
        n1290 = property on="Report" class="Bool (strict)"("DisabledEnum"=w1194) -> ()  [unwired: 2 in, 2 out]
        n1291 = property on="Test Setup" class="Bool (strict)"("DisabledEnum"=w1194) -> ()  [unwired: 2 in, 2 out]
        n1292 = case shown="True" w1193 {
          tunnel: [T18."Disabled" ("Disabled") T18."Enabled" ("Disabled")] -> w1192
          frame False {
          }
          frame True {
          }
        }
        n1293 = property on="About" class="Bool (strict)"("DisabledEnum"=w1192) -> ()  [unwired: 2 in, 2 out]
      }
      frame "Adv Scar" {
        w1201 = T18."Enabled" ("Disabled")
        n1294 = property on="Dashboard" class="Bool (strict)"("DisabledEnum"=T18."Disabled" ("Disabled")) -> ()  [unwired: 2 in, 2 out]
        n1295 = property on="Imaging" class="Bool (strict)"("DisabledEnum"=w1201) -> ()  [unwired: 2 in, 2 out]
        n1296 = property on="Analysis" class="Bool (strict)"("DisabledEnum"=w1201) -> ()  [unwired: 2 in, 2 out]
        n1297 = property on="Home" class="Bool (strict)"("DisabledEnum"=w1201) -> ()  [unwired: 2 in, 2 out]
        n1298 = property on="Report" class="Bool (strict)"("DisabledEnum"=w1201) -> ()  [unwired: 2 in, 2 out]
        n1299 = property on="Test Setup" class="Bool (strict)"("DisabledEnum"=w1201) -> ()  [unwired: 2 in, 2 out]
        n1300 = local read "Service Password enable"() -> (w1199:bool)
        n1301 = case shown="True" w1199 {
          tunnel: [T18."Disabled" ("Disabled") T18."Enabled" ("Disabled")] -> w1198
          frame False {
          }
          frame True {
          }
        }
        n1302 = property on="About" class="Bool (strict)"("DisabledEnum"=w1198) -> ()  [unwired: 2 in, 2 out]
      }
      frame "Calibration" {
        w1204 = T18."Enabled" ("Disabled")
        n1303 = property on="Dashboard" class="Bool (strict)"("DisabledEnum"=T18."Disabled" ("Disabled")) -> ()  [unwired: 2 in, 2 out]
        n1304 = property on="Imaging" class="Bool (strict)"("DisabledEnum"=w1204) -> ()  [unwired: 2 in, 2 out]
        n1305 = property on="Analysis" class="Bool (strict)"("DisabledEnum"=w1204) -> ()  [unwired: 2 in, 2 out]
        n1306 = property on="Home" class="Bool (strict)"("DisabledEnum"=w1204) -> ()  [unwired: 2 in, 2 out]
        n1307 = property on="Report" class="Bool (strict)"("DisabledEnum"=w1204) -> ()  [unwired: 2 in, 2 out]
        n1308 = property on="Test Setup" class="Bool (strict)"("DisabledEnum"=w1204) -> ()  [unwired: 2 in, 2 out]
        n1309 = local read "Service Password enable"() -> (w1206:bool)
        n1310 = property on="Calibration" class="Bool (strict)"("DisabledEnum"=w1204) -> ()  [unwired: 2 in, 2 out]
        n1311 = case shown="True" w1206 {
          tunnel: [T18."Disabled" ("Disabled") T18."Enabled" ("Disabled")] -> w1205
          frame False {
          }
          frame True {
          }
        }
        n1312 = property on="About" class="Bool (strict)"("DisabledEnum"=w1205) -> ()  [unwired: 2 in, 2 out]
      }
      frame "Adv Scar Report" {
        w1212 = T18."Enabled" ("Disabled")
        n1313 = property on="Dashboard" class="Bool (strict)"("DisabledEnum"=T18."Disabled" ("Disabled")) -> ()  [unwired: 2 in, 2 out]
        n1314 = property on="Imaging" class="Bool (strict)"("DisabledEnum"=w1212) -> ()  [unwired: 2 in, 2 out]
        n1315 = property on="Analysis" class="Bool (strict)"("DisabledEnum"=w1212) -> ()  [unwired: 2 in, 2 out]
        n1316 = property on="Home" class="Bool (strict)"("DisabledEnum"=w1212) -> ()  [unwired: 2 in, 2 out]
        n1317 = property on="Report" class="Bool (strict)"("DisabledEnum"=w1212) -> ()  [unwired: 2 in, 2 out]
        n1318 = property on="Test Setup" class="Bool (strict)"("DisabledEnum"=w1212) -> ()  [unwired: 2 in, 2 out]
        n1319 = local read "Service Password enable"() -> (w1211:bool)
        n1320 = case shown="True" w1211 {
          tunnel: [T18."Disabled" ("Disabled") T18."Enabled" ("Disabled")] -> w1210
          frame False {
          }
          frame True {
          }
        }
        n1321 = property on="About" class="Bool (strict)"("DisabledEnum"=w1210) -> ()  [unwired: 2 in, 2 out]
      }
      frame "Compare Files" {
        w1218 = T18."Enabled" ("Disabled")
        n1322 = local read "Service Password enable"() -> (w1217:bool)
        n1323 = property on="Dashboard" class="Bool (strict)"("DisabledEnum"=T18."Disabled" ("Disabled")) -> ()  [unwired: 2 in, 2 out]
        n1324 = property on="Imaging" class="Bool (strict)"("DisabledEnum"=w1218) -> ()  [unwired: 2 in, 2 out]
        n1325 = property on="Analysis" class="Bool (strict)"("DisabledEnum"=w1218) -> ()  [unwired: 2 in, 2 out]
        n1326 = property on="Home" class="Bool (strict)"("DisabledEnum"=w1218) -> ()  [unwired: 2 in, 2 out]
        n1327 = property on="Report" class="Bool (strict)"("DisabledEnum"=w1218) -> ()  [unwired: 2 in, 2 out]
        n1328 = property on="Test Setup" class="Bool (strict)"("DisabledEnum"=w1218) -> ()  [unwired: 2 in, 2 out]
        n1329 = case shown="True" w1217 {
          tunnel: [T18."Disabled" ("Disabled") T18."Enabled" ("Disabled")] -> w1216
          frame False {
          }
          frame True {
          }
        }
        n1330 = property on="About" class="Bool (strict)"("DisabledEnum"=w1216) -> ()  [unwired: 2 in, 2 out]
      }
      frame "Acquire" {
        n1331 = local read "Service Password enable"() -> (w1223:bool)
        n1332 = property on="Test Setup" class="Bool (strict)"("DisabledEnum"=T18."Disabled" ("Disabled")) -> ()  [unwired: 2 in, 2 out]
        n1333 = local read "Auto Start Test"() -> (w1225:bool)
        n1334 = local read "RUN"() -> (w1227:bool)
        n1335 = case shown="True" w1223 {
          tunnel: [T18."Disabled" ("Disabled") T18."Enabled" ("Disabled")] -> w1224
          frame False {
          }
          frame True {
          }
        }
        n1336 = Or(x=w1227, y=w1225) -> (x .or. y?=w1226:bool)
        n1337 = case shown="True" w1226 {
          tunnel: [T18."Enabled" ("Disabled") T18."Disabled" ("Disabled")] -> w1222
          frame False {
          }
          frame True {
          }
        }
        n1338 = property on="About" class="Bool (strict)"("DisabledEnum"=w1224) -> ()  [unwired: 2 in, 2 out]
        n1339 = property on="Imaging" class="Bool (strict)"("DisabledEnum"=w1222) -> ()  [unwired: 2 in, 2 out]
        n1340 = property on="Dashboard" class="Bool (strict)"("DisabledEnum"=w1222) -> ()  [unwired: 2 in, 2 out]
        n1341 = property on="Analysis" class="Bool (strict)"("DisabledEnum"=w1222) -> ()  [unwired: 2 in, 2 out]
        n1342 = property on="Home" class="Bool (strict)"("DisabledEnum"=w1222) -> ()  [unwired: 2 in, 2 out]
        n1343 = property on="Report" class="Bool (strict)"("DisabledEnum"=w1222) -> ()  [unwired: 2 in, 2 out]
        n1344 = property on="Calibration" class="Bool (strict)"("DisabledEnum"=w1222) -> ()  [unwired: 2 in, 2 out]
      }
      frame "About" {
        n1345 = local read "FILE"() -> (w1241:string)
        n1346 = local read "TEST FILE NAM,E SAVED"() -> (w1234:bool)
        n1347 = call <vilib>:"Trim Whitespace.vi"("string"=w1241) -> ("trimmed string"=w1240:string)  [unwired: 1 in]
        n1348 = local read "Auto Start Test"() -> (w1244:bool)
        n1349 = String Length(string=w1240) -> (length=w1239:i32)
        n1350 = Greater?(x=w1239, y=1) -> (0:w1236:bool)
        n1351 = And(x=w1236, y=w1234) -> (x .and. y?=w1235:bool)
        n1352 = local read "RUN"() -> (w1246:bool)
        n1353 = case shown="True" w1235 {
          tunnel: [T18."Disabled" ("Disabled") T18."Enabled" ("Disabled")] -> w1237
          frame False {
          }
          frame True {
          }
        }
        n1354 = Or(x=w1246, y=w1244) -> (x .or. y?=w1245:bool)
        n1355 = property on="About" class="Bool (strict)"("DisabledEnum"=T18."Enabled" ("Disabled")) -> ()  [unwired: 2 in, 2 out]
        n1356 = case shown="False" w1245 {
          tunnel: [T18."Enabled" ("Disabled") T18."Disabled" ("Disabled")] -> w1243
          frame False {
          }
          frame True {
          }
        }
        n1357 = property on="Dashboard" class="Bool (strict)"("DisabledEnum"=w1237) -> ()  [unwired: 2 in, 2 out]
        n1358 = property on="Test Setup" class="Bool (strict)"("DisabledEnum"=T18."Disabled" ("Disabled")) -> ()  [unwired: 2 in, 2 out]
        n1359 = property on="Imaging" class="Bool (strict)"("DisabledEnum"=w1243) -> ()  [unwired: 2 in, 2 out]
        n1360 = property on="Analysis" class="Bool (strict)"("DisabledEnum"=w1243) -> ()  [unwired: 2 in, 2 out]
        n1361 = property on="Home" class="Bool (strict)"("DisabledEnum"=w1243) -> ()  [unwired: 2 in, 2 out]
        n1362 = property on="Report" class="Bool (strict)"("DisabledEnum"=w1243) -> ()  [unwired: 2 in, 2 out]
      }
    }
    n1363 = local read "Quit"() -> (w1171:bool)
    "Single" <- "Single - Graph"
  }
  n1364 = disable-structure shown="Disabled" {
    disable-tunnel: [w1523 _] -> w39
    disable-tunnel: _ -> [w1522 _]
    frame Disabled {
      n1365 = while {
        tunnel: w1522 -> [_]
        tunnel: [w1524] -> w1523
        tunnel: [w1525] -> _
        i -> [w1525]
        stop <- w1524 stop-if-true
        w1541 = u16 10 items=["1.0"=10, "1.5"=15, "2.0"=20] ("stop bits (10: 1 bit)")
        n1366 = Wait (ms)(milliseconds to wait=u32 10) -> ()  [unwired: 1 out]
        n1367 = call-poly "VISA Configure Serial Port"("VISA resource name"=refnum<visa-resource-name> "ASRL1::INSTR" ("COM PORT"), "timeout (10sec)"=u32 10, "baud rate (9600)"=u32 57600, "data bits (8)"=u16 8, "stop bits (10: 1 bit)"=w1541) -> ("VISA resource name out"=w1527:refnum<visa-resource-name>, "error out"=w1536:errorcluster)  [unwired: 9 in]
        n1368 = VISA Read(VISA resource name=w1527, byte count=u32 2 ("byte count (0)")) -> (read buffer=w1535:string)  [unwired: 1 in, 3 out]
        n1369 = String Subset(string=w1535, offset (0)=0, length (rest)=2 ("length (rest)")) -> (substring=w1534:string)
        n1370 = Match Pattern(string=w1534, regular expression="<>") -> (offset past match=w1531:i32)  [unwired: 1 in, 3 out]
        n1371 = Greater Or Equal?(x=w1531, y=0) -> (x >= y?=w1526:bool)
        n1372 = case shown="True" w1526 {
          tunnel: w1527 -> [_ w1545]
          tunnel: w1536 -> [_ w1544]
          frame False {
          }
          frame True {
            n1373 = VISA Read(VISA resource name=w1545, byte count=u32 32 ("byte count (0)"), error in (no error)=w1544) -> (read buffer=w1543:string)  [unwired: 3 out]
            n1374 = String Subset(string=w1543, offset (0)=0, length (rest)=8 ("length (rest)")) -> (substring=w1547:string)
            n1375 = String Subset(string=w1543, offset (0)=8, length (rest)=8 ("length (rest)")) -> (substring=w1548:string)
            n1376 = Decimal String To Number(string=w1548) -> (number=w1555:i32)  [unwired: 2 in, 1 out]
            n1377 = Decimal String To Number(string=w1547) -> (number=w1551:i32)  [unwired: 2 in, 1 out]
            n1378 = Divide(x=w1555, y=10000) -> ()  [unwired: 1 out]
            n1379 = Divide(x=w1551, y=1000000) -> ()  [unwired: 1 out]
          }
        }
        n1380 = local read "Quit"() -> (w1524:bool)
      }
    }
    frame Enabled {
    }
  }
  n1381 = while {
    shift-right: [w1570] -> w52
    shift-left: _ -> [w1561]
    shift-right: [w1569] -> w51
    shift-left: errorcluster {"status"=TRUE, "code"=0, "source"="Init"} ("error IO") -> [w1563]
    tunnel: [w1558] -> w42
    tunnel: [w1568] -> _
    i -> [w1568]
    stop <- w1558 stop-if-true
    n1382 = local read "Port 1a"() -> (w1564:bool)
    n1383 = local read "Port 3"() -> (w1565:bool)
    n1384 = local read "Com Port 1"() -> (w1562:refnum<visa-resource-name>)
    n1385 = Or(x=w1565, y=w1564) -> (x .or. y?=w1567:bool)
    n1386 = Unbundle(w1563) -> ("status"=→"Port 3":bool)  [unwired: 2 out]
    n1387 = Not Equal?(x=w1562, y=w1561) -> (x != y?=w1559:bool)
    n1388 = case shown="True" w1567 {
      frame False {
        w1573 = TRUE ("Visible")
        n1389 = property on="Port 1a" class="Bool (strict)"("Visible"=w1573) -> ()  [unwired: 2 in, 2 out]
        n1390 = property on="Port 3" class="Bool (strict)"("Visible"=w1573) -> ()  [unwired: 2 in, 2 out]
      }
      frame True {
        w1574 = TRUE ("Visible")
        n1391 = property on="Port 1a" class="Bool (strict)"("Visible"=w1574) -> ()  [unwired: 2 in, 2 out]
        n1392 = property on="Port 3" class="Bool (strict)"("Visible"=w1574) -> ()  [unwired: 2 in, 2 out]
      }
    }
    n1393 = Wait (ms)(milliseconds to wait=u32 40) -> ()  [unwired: 1 out]
    n1394 = case shown="True" w1559 {
      tunnel: [w1571 errorcluster {"status"=TRUE, "code"=0, "source"="Init"} ("error out")] -> w1560
      tunnel: w1563 -> [w1571 _]
      frame False {
      }
      frame True {
      }
    }
    n1395 = case shown="Error" w1560 {
      selector: w1560 -> [w1582 w1609]
      tunnel: [w1576 w1613] -> w1570
      tunnel: [w1584 w1607] -> w1569
      tunnel: w1561 -> [w1583 w1611]
      frame No Error {
        n1396 = property class="Instr"(reference=w1583, error in=w1582) -> (reference out=w1580:refnum<visa-resource-name>, error out=w1581:errorcluster, "Serial Settings:Number of Bytes at Serial Port"=w1577:u32)
        n1397 = Greater?(x=w1577, y=u32 5) -> (0:w1575:bool)
        n1398 = Not(x=w1575) -> (.not. x?=→"Port 1a":bool)
        n1399 = while {
          tunnel: [w1602] -> w1584
          tunnel: [w1601] -> w1585
          tunnel: w1581 -> [w1600]
          tunnel: w1580 -> [w1599]
          stop <- TRUE stop-if-true
          n1400 = property class="Instr" props=["Serial Settings:Number of Bytes at Serial Port"](reference=w1599, error in=w1600) -> (reference out=w1604:refnum<visa-resource-name>, error out=w1603:errorcluster)  [unwired: 1 out]
          n1401 = VISA Read(VISA resource name=w1604, byte count=u32 50, error in (no error)=w1603) -> (VISA resource name out=w1601:refnum<visa-resource-name>, read buffer=w1586:string, error out=w1602:errorcluster)  [unwired: 1 out]
          "UNI READ" <- w1586
          n1402 = Spreadsheet String To Array(delimiter (Tab)=";", format string="", spreadsheet string=w1586, array type (2D Dbl)=dbl[] []) -> (array=w1596:dbl[])
          n1403 = Index Array(array=w1596) -> (element #1=→"LVDT MIN":dbl, element #2=→"LVDT MAX":dbl, element #3=→"LVDT Peak":dbl, element #4=→"pizo raw":dbl, element #5=→"Friction":dbl, element #6=→"cof 2":dbl)  [unwired: 6 in]
        }
        n1404 = VISA Flush I/O Buffer(VISA resource name=w1585) -> (VISA resource name out=w1576:refnum<visa-resource-name>)  [unwired: 2 in, 1 out]
      }
      frame Error {
        w1619 = u16 0 items=["None", "XON/XOFF", "RTS/CTS", "XON/XOFF & RTS/CTS", "DTR/DSR", "XON/XOFF & DTR/DSR"] ("flow control (0:none)  2")
        w1617 = u16 10 items=["1.0"=10, "1.5"=15, "2.0"=20] ("stop bits 2")
        w1615 = u16 0 items=["None", "Odd", "Even", "Mark", "Space"] ("parity 2")
        w1616 = u32 10000  # timeout (10sec)
        n1405 = VISA Close(VISA resource name=w1611, error in (no error)=w1609) -> (error out=w1612:errorcluster)
        n1406 = local write "Port 1a"(FALSE ("Port 1a")) -> ()
        n1407 = local read "Com Port 1"() -> (w1606:refnum<visa-resource-name>)
        n1408 = call <vilib>:"Clear Errors.vi"("error in (no error)"=w1612) -> ("error out"=w1610:errorcluster)  [unwired: 5 in, 1 out]
        n1409 = call-poly "VISA Configure Serial Port"("VISA resource name"=w1606, "timeout (10sec)"=w1616, "baud rate (9600)"=u32 250000 ("baud rate  2"), "data bits (8)"=u16 8 ("data bits  2"), "parity (0:none)"=w1615, "error in (no error)"=w1610, "stop bits (10: 1 bit)"=w1617, "flow control (0:none)"=w1619) -> ("VISA resource name out"=w1620:refnum<visa-resource-name>, "error out"=w1621:errorcluster)  [unwired: 6 in]
        n1410 = flat-sequence {
          tunnel: w1620 -> [w1623]
          tunnel: w1621 -> [w1622]
          tunnel: [w1623] -> w1613
          tunnel: [w1622] -> w1607
          frame #0 {
            n1411 = Wait (ms)(milliseconds to wait=u32 50) -> ()  [unwired: 1 out]
          }
        }
        "Residual Uno" <- ""
        "Port 1 Error" <- w1607
      }
    }
    n1412 = local read "Quit"() -> (w1558:bool)
    "Error Uno" <- w1563
  }
  n1413 = while {
    stop <- w1633 stop-if-true
    # "V0OLTAGE TO STROKE (peice vise calibration)"
    n1414 = Wait (ms)(milliseconds to wait=u32 10) -> ()  [unwired: 1 out]
    n1415 = local read "LVDT Peak"() -> (w1625:dbl)
    n1416 = formula code="// Dynamic Parameterized Linear Interpolation Node\n// Inputs: vpp_val, voltages (Array), distances (Array)\n// Outputs: stroke\n\nint i = 0;\nint segments = 11; // 12 points make 11 interpolation segments\n\n// 1. Lower Boundary Clamp\nif (vpp_val <= voltages[0]) {\n    stroke = distances[0];\n}\n// 2. Upper Boundary Clamp\nelse if (vpp_val >= voltages[segments]) {\n    stroke = distances[segments];\n}\n// 3. Dynamic Segment Search Loop\nelse {\n    stroke = distances[0]; // Fallback baseline\n    for (i = 0; i < segments; i++) {\n        if (vpp_val >= voltages[i] && vpp_val <= voltages[i+1]) {\n            // Standard linear interpolation formula using array lookups\n            stroke = distances[i] + (vpp_val - voltages[i]) * (distances[i+1] - distances[i]) / (voltages[i+1] - voltages[i]);\n            break; // Segment found, safely exit the loop\n        }\n    }\n}"("vpp_val"=w1625, "voltages"="calibration values", "distances"="STROKE") -> ("stroke"=→"LVDT STROKE":dbl)
    n1417 = local read "Calibration Tare Value"() -> (w1629:dbl)
    n1418 = local read "Calibration Tare"() -> (w1627:bool)
    n1419 = Subtract(x=w1625, y=w1629) -> (x-y=→"LVDT STROKE  Calibration":dbl)
    n1420 = case shown="True" w1627 {
      selector: w1627 -> [_ w1635]
      tunnel: w1625 -> [_ w1636]
      frame False {
      }
      frame True {
        n1421 = Not(x=w1635) -> (.not. x?=w1634:bool)
        n1422 = local write "Calibration Tare"(w1634) -> ()
        "Calibration Tare Value" <- w1636
      }
    }
    n1423 = local read "Quit"() -> (w1633:bool)
  }
  n1424 = while {
    stop <- w1656 stop-if-true
    n1425 = call <vilib>:"High Resolution Polling Wait.vi"("seconds to wait"=0.02) -> ()  [unwired: 10 in, 1 out]
    n1426 = local read "Due read"() -> (w1654:string)
    n1427 = Spreadsheet String To Array(delimiter (Tab)=";", format string="", spreadsheet string=w1654, array type (2D Dbl)=string[] []) -> (array=w1651:string[])
    n1428 = Fract/Exp String To Number(string=w1651) -> (number=w1650:dbl[])  [unwired: 3 in, 1 out]
    n1429 = Index Array(array=w1650) -> (element #1=→"Sample Temperature":dbl, element #2=→"Target Sample Temperature":dbl, element #3=→"Current Duty Cycle":dbl, element #4=→"Ambient Temperature":dbl, element #5=→"Dac Status":dbl, element #6=→"Vpp":dbl, element #7=→"Active Error Code":dbl, element #8=→"Kp":dbl, element #9=→"Ki":dbl, element #10=→"Kd":dbl, element #11=→"SampleRaw":dbl, element #12=→"AmbRaw":dbl)  [unwired: 12 in]
    n1430 = local read "Quit"() -> (w1656:bool)
  }
  n1431 = while {
    shift-right: [w1670] -> w37
    shift-left: _ -> [w1661]
    shift-right: [w1669] -> w36
    shift-left: errorcluster {"status"=FALSE, "code"=0, "source"="Init"} ("error out") -> [w1663]
    tunnel: [w1658] -> w41
    tunnel: [w1668] -> _
    i -> [w1668]
    stop <- w1658 stop-if-true
    n1432 = local read "Com Port 2"() -> (w1662:refnum<visa-resource-name>)
    n1433 = local read "Port 2a"() -> (w1664:bool)
    n1434 = Unbundle(w1663) -> ("status"=→"Port 4":bool)  [unwired: 2 out]
    n1435 = call <vilib>:"High Resolution Polling Wait.vi"("seconds to wait"=0.02) -> ()  [unwired: 10 in, 1 out]
    n1436 = local read "Port 4"() -> (w1665:bool)
    n1437 = Not Equal?(x=w1662, y=w1661) -> (x != y?=w1660:bool)
    n1438 = Or(x=w1665, y=w1664) -> (x .or. y?=w1667:bool)
    n1439 = case shown="False" w1667 {
      frame False {
        w1673 = TRUE ("Visible")
        n1440 = property on="Port 2a" class="Bool (strict)"("Visible"=w1673) -> ()  [unwired: 2 in, 2 out]
        n1441 = property on="Port 4" class="Bool (strict)"("Visible"=w1673) -> ()  [unwired: 2 in, 2 out]
      }
      frame True {
        w1674 = TRUE ("Visible")
        n1442 = property on="Port 2a" class="Bool (strict)"("Visible"=w1674) -> ()  [unwired: 2 in, 2 out]
        n1443 = property on="Port 4" class="Bool (strict)"("Visible"=w1674) -> ()  [unwired: 2 in, 2 out]
      }
    }
    n1444 = case shown="True" w1660 {
      tunnel: [w1671 errorcluster {"status"=TRUE, "code"=0, "source"="Init"} ("error out")] -> w1659
      tunnel: w1663 -> [w1671 _]
      frame False {
      }
      frame True {
      }
    }
    n1445 = case shown="Error" w1659 {
      selector: w1659 -> [w1686 w1718]
      tunnel: [w1679 w1723] -> w1670
      tunnel: [w1687 w1716] -> w1669
      tunnel: w1661 -> [w1689 w1721]
      frame No Error {
        n1446 = property class="Instr" props=["Serial Settings:Number of Bytes at Serial Port"](reference=w1689, error in=w1686) -> (reference out=w1680:refnum<visa-resource-name>, error out=w1685:errorcluster)  [unwired: 1 out]
        n1447 = while {
          tunnel: [w1697] -> w1681
          tunnel: [w1696] -> w1682
          tunnel: w1685 -> [w1695]
          tunnel: w1680 -> [w1694]
          tunnel: [w1693] -> _
          i -> [w1693]
          stop <- TRUE stop-if-true
          n1448 = property class="Instr" props=["Serial Settings:Number of Bytes at Serial Port"](reference=w1694, error in=w1695) -> (reference out=w1699:refnum<visa-resource-name>, error out=w1698:errorcluster)  [unwired: 1 out]
          n1449 = VISA Read(VISA resource name=w1699, byte count=u32 1000, error in (no error)=w1698) -> (VISA resource name out=w1696:refnum<visa-resource-name>, read buffer=→"Due read":string, error out=w1697:errorcluster)  [unwired: 1 out]
        }
        n1450 = local read "Command"() -> (w1677:string)
        n1451 = call <vilib>:"Trim Whitespace.vi"("string"=w1677) -> ("trimmed string"=w1676:string)  [unwired: 1 in]
        n1452 = Not Equal?(x=w1676, y="") -> (x != y?=w1683:bool)
        n1453 = case shown="True" w1683 {
          tunnel: w1682 -> [w1701 w1706]
          tunnel: [w1701 w1710] -> w1688
          tunnel: w1681 -> [w1700 w1705]
          tunnel: [w1700 w1708] -> w1687
          tunnel: w1676 -> [_ w1704]
          tunnel: [_ w1707] -> _
          frame False {
            # "DATA  WRITE LOOP"
          }
          frame True {
            n1454 = Concatenate Strings(w1704, "\r\n") -> (w1703:string)
            n1455 = VISA Write(VISA resource name=w1706, write buffer=w1703, error in (no error)=w1705) -> (VISA resource name out=w1710:refnum<visa-resource-name>, return count=w1707:u32, error out=w1709:errorcluster)
            n1456 = flat-sequence {
              tunnel: w1709 -> [w1712]
              tunnel: [w1712] -> w1708
              frame #0 {
                n1457 = local write "Command"("" ("Command")) -> ()
                n1458 = Wait (ms)(milliseconds to wait=u32 5) -> ()  [unwired: 1 out]
              }
